vi "Constrain.vi"(10 "Particle.lvclass":refnum<class "Particle.lvclass">, 11 "World in":refnum<class "World.lvclass">) -> (2 "Particle":refnum<class "Particle.lvclass">, 3 "World out":refnum<class "World.lvclass">)   [LabVIEW 2020, in "World.lvclass"]
uses:
  World.lvclass
  Particle.lvclass
  Particle/Position.ctl
  World.lvclass/World.ctl
  Particle.lvclass/Particle.ctl
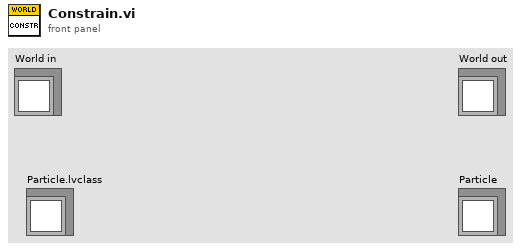
[diagram p1: front panel]
types:
  T1 = typedef "Particle.lvclass/Position.ctl" = cluster{"X":i32, "Y":i32}
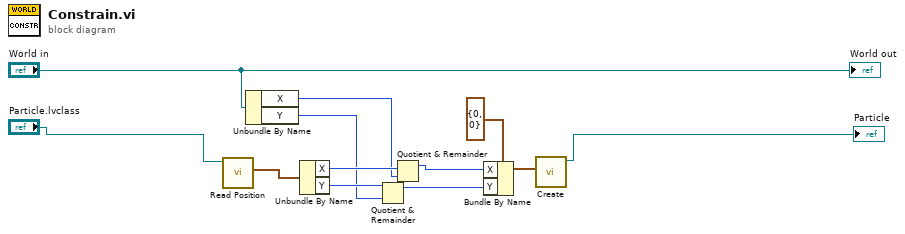
[diagram p0: block diagram]
diagram:
  n1 = call "Read Position.vi"("Particle in"="Particle.lvclass") -> ("Position"=w12:T1)  [unwired: 10 in]
  n2 = Unbundle By Name("World in") -> ("X"=w5:i32, "Y"=w1:i32)
  n3 = Unbundle By Name(w12) -> ("X"=w6:i32, "Y"=w3:i32)
  n4 = Quotient & Remainder(x=w3, y=w1) -> (x-y*floor(x/y)=w2:i32)  [unwired: 1 out]
  n5 = Quotient & Remainder(x=w6, y=w5) -> (x-y*floor(x/y)=w4:i32)  [unwired: 1 out]
  n6 = Bundle By Name(cluster=T1 {"X"=0, "Y"=0} ("Position"), "X"=w4, "Y"=w2) -> (w9:T1)
  n7 = call "Create.vi"("Position"=w9) -> ("Particle out"=→"Particle":refnum<class "Particle.lvclass">)  [unwired: 10 in]
  "World out" <- "World in"
